vi "Utility folder.vi"(9 "Action":T1) -> (1 "Output":string)   [LabVIEW 2015, in "NIVS_Consolidated_CDW_MetaDataObj.lvclass"]
doc: "Constants, which are necessary for the virtual folder <B>Utility</B> in the generated custom device project."
uses:
  NIVS_Consolidated_CDW_MetaDataObj.lvclass
  Utility folder.ctl
  Common.ctl
  Common.vi
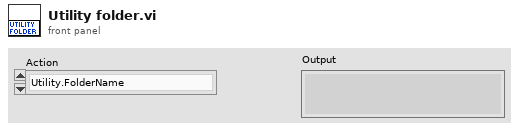
[diagram p1: front panel]
types:
  T1 = typedef "NIVS_Consolidated_CDW_MetaDataObj.lvclass/Utility folder.ctl" = enum16{"Utility.FolderName", "Utility.Copy .llb to NI VeriStand dir.FileName", "Utility.Copy .llb to NI VeriStand dir.FilePathAndName", "Utility.LLB Pre Build.FilePathAndName"}
  T2 = typedef "NIVS_Consolidated_CDW_MetaDataObj.lvclass/Common.ctl" = enum16{"ProjectName", "TemplatesFolderName", "ProjectTemplatePathAndName", "TimingAndSyncFolderName", "CustomDeviceFolderName", "PathToTemplates"}
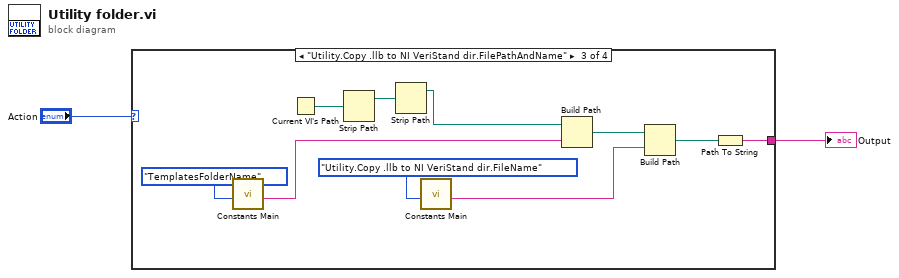
[diagram p0: block diagram]
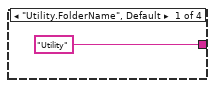
[diagram p2: hidden frame]
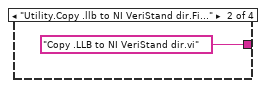
[diagram p3: hidden frame]
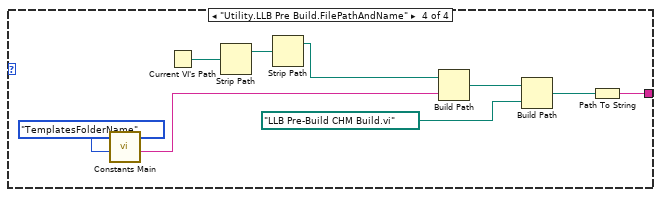
[diagram p4: hidden frame]
diagram:
  n1 = case shown="\"Utility.Copy .llb to NI VeriStand dir.FilePathAndName\"" "Action" {
    tunnel: ["Utility" "Copy .LLB to NI VeriStand dir.vi" ("name or relative path") w11 w20] -> w1
    frame "Utility.FolderName", Default {
    }
    frame "Utility.Copy .llb to NI VeriStand dir.FileName" {
    }
    frame "Utility.Copy .llb to NI VeriStand dir.FilePathAndName" {
      n2 = call-poly "Constants Main.vi"("Action"=Common."TemplatesFolderName") -> ("Output"=w14:string)  [unwired: 10 in]
      n3 = Current VI's Path() -> (path=w7:path)
      n4 = Strip Path(path=w7) -> (stripped path=w6:path)  [unwired: 1 out]
      n5 = Strip Path(path=w6) -> (stripped path=w5:path)  [unwired: 1 out]
      n6 = call-poly "Constants Main.vi"("Action"=Utility_folder."Utility.Copy .llb to NI VeriStand dir.FileName") -> ("Output"=w8:string)  [unwired: 10 in]
      n7 = Build Path(base path=w5, name or relative path=w14) -> (appended path=w13:path)
      n8 = Build Path(base path=w13, name or relative path=w8) -> (appended path=w10:path)
      n9 = Path To String(path=w10) -> (string=w11:string)
    }
    frame "Utility.LLB Pre Build.FilePathAndName" {
      n10 = call-poly "Constants Main.vi"("Action"=Common."TemplatesFolderName") -> ("Output"=w23:string)  [unwired: 10 in]
      n11 = Current VI's Path() -> (path=w18:path)
      n12 = Strip Path(path=w18) -> (stripped path=w17:path)  [unwired: 1 out]
      n13 = Strip Path(path=w17) -> (stripped path=w16:path)  [unwired: 1 out]
      n14 = Build Path(base path=w16, name or relative path=w23) -> (appended path=w22:path)
      n15 = Build Path(base path=w22, name or relative path=path "LLB Pre-Build CHM Build.vi") -> (appended path=w19:path)
      n16 = Path To String(path=w19) -> (string=w20:string)
    }
  }
  "Output" <- w1
